vi "image_encode_base64.vi"(2 "error in (no error)":errorcluster, 3 "imagepaths":path[](array[path])) -> (0 "error out":errorcluster, 1 "image_data":string[](array[string]))   [LabVIEW 2020, in "llm_openai_chatmodels.lvclass"]
uses:
  llm_openai_chatmodels.lvclass
  <vilib>/httpClient/LabVIEWHTTPClient.lvlib
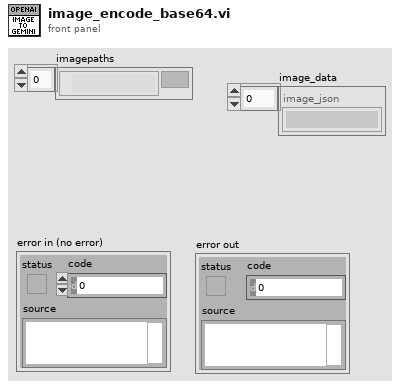
[diagram p1: front panel]
types:
  T1 = cluster{"type":string, "image_url":cluster{"url":string}}
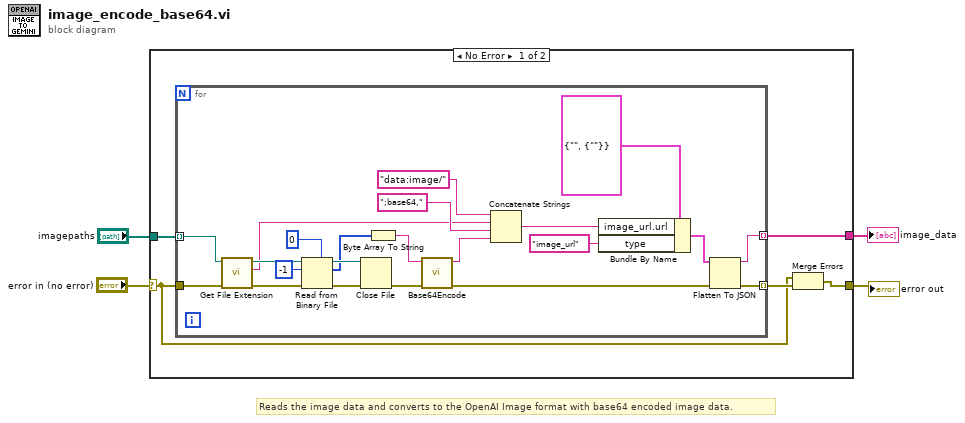
[diagram p0: block diagram]
diagram:
  # "Reads the image data and converts to the OpenAI Image format with base64 encoded image data."
  n1 = case shown="No Error" "error in (no error)" {
    selector: "error in (no error)" -> [w5 w32]
    tunnel: [w9 _] -> w4
    tunnel: "imagepaths" -> [w8 _]
    tunnel: [w6 w32] -> w2
    frame No Error {
      n2 = for {
        tunnel: [w21] -> w9 mode=indexing
        tunnel: w8 -> [w25] mode=indexing
        tunnel: [w23] -> w7 mode=indexing
        tunnel: w5 -> [w24]
        n3 = call <vilib>:"Get File Extension.vi"("error in (no error)"=w24, "file"=w25) -> ("error out"=w31:errorcluster, "lowercase file extension"=w13:string, "dup file"=w30:path)  [unwired: 5 in, 2 out]
        n4 = Read from Binary File(5:u8 0 ("unsigned 8bit integer"), 8:w31, 10:-1 ("count (1)"), 11:w30) -> (0:w28:errorcluster, 2:w19:u8[], 3:w29:refnum<file>)  [unwired: 2 in, 1 out]
        n5 = Close File(refnum=w29, error in=w28) -> (error out=w18:errorcluster)  [unwired: 1 out]
        n6 = Byte Array To String(unsigned byte array=w19) -> (string=w20:string)
        n7 = call <vilib>:"Base64Encode.vi"("error in (no error)"=w18, "buffer in"=w20) -> ("error out"=w17:errorcluster, "encoded string"=w12:string)  [unwired: 8 in]
        n8 = Concatenate Strings("data:image/" ("string"), w13, ";base64," ("string"), w12) -> (w11:string)
        n9 = Bundle By Name(cluster=T1 {"type"="", "image_url"={"url"=""}} ("content"), "image_url.url"=w11, "type"="image_url") -> (w22:T1)
        n10 = Flatten To JSON(anything=w22, error in (no error)=w17) -> (JSON string=w21:string, 11:w23:errorcluster)  [unwired: 1 in]
      }
      n11 = Merge Errors(w5, w7) -> (w6:errorcluster)
    }
    frame Error {
    }
  }
  "image_data" <- w4
  "error out" <- w2
